vi "getSavePath.vi"(0 "beam_name":string, 5 "Polarizer":string, 7 "Analyzer":string(combo), 9 "prefix":string, 11 "suffix":string, 12 "active":u16) -> (4 "appended filename":string)   [LabVIEW 2023]
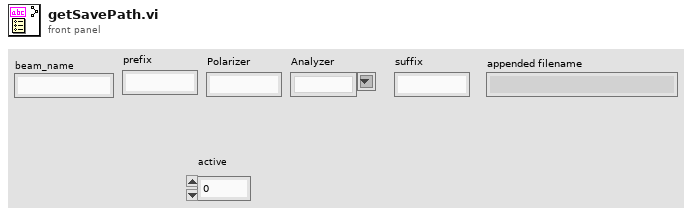
[diagram p1: front panel]
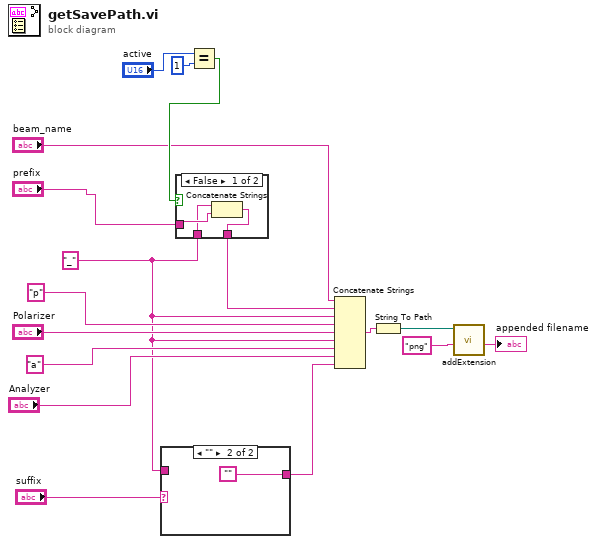
[diagram p0: block diagram]
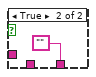
[diagram p2: hidden frame]
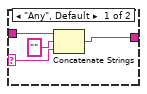
[diagram p3: hidden frame]
diagram:
  w1 = "_" ("string")
  n1 = case shown="\"\"" "suffix" {
    selector: "suffix" -> [w19 _]
    tunnel: w1 -> [w21 _]
    tunnel: [w18 ""] -> w17
    frame "Any", Default {
      n2 = Concatenate Strings(w21, "" ("string"), w19) -> (w18:string)
    }
    frame "" {
    }
  }
  n3 = Equal?(x="active", y=u16 1) -> (x = y?=w5:bool)
  n4 = case shown="False" w5 {
    tunnel: [w23 ""] -> w4
    tunnel: "prefix" -> [w25 _]
    tunnel: w1 -> [w24 _]
    frame False {
      n5 = Concatenate Strings(w24, w25) -> (w23:string)
    }
    frame True {
    }
  }
  n6 = Concatenate Strings("beam_name", w4, w1, "p" ("string"), "Polarizer", w1, "a" ("string"), "Analyzer", w17) -> (w12:string)
  n7 = String To Path(string=w12) -> (path=w13:path)
  n8 = call "addExtension.vi"("Extension"="png" ("pattern label"), "In path"=w13) -> ("Out path"=→"appended filename":string)  [unwired: 8 in, 1 out]
